vi "Scale.vi"(8 "Offset":dbl, 9 "Factor":dbl=1.0, 10 "FullScale":dbl=1.0, 11 "Input":dbl) -> (3 "Output":dbl)   [LabVIEW 2011]
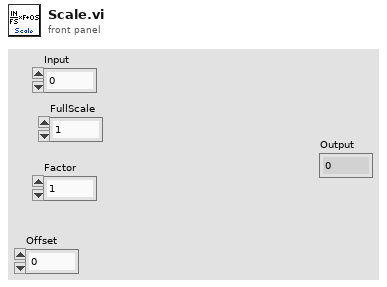
[diagram p1: front panel]
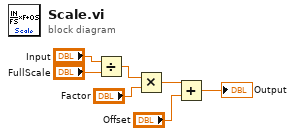
[diagram p0: block diagram]
diagram:
  n1 = Divide(x="Input", y="FullScale") -> (x/y=w5:dbl)
  n2 = Multiply(x=w5, y="Factor") -> (x*y=w3:dbl)
  n3 = Add(x=w3, y="Offset") -> (x+y=→"Output":dbl)
